vi "Tabelle zerlegen.vi"(11 "Tabelle":string[][](array[string])) -> (0 "Text":string[](array[string]), 1 "abschaltend":bool[](array[boolean]), 2 "quittieren?":bool[](array[boolean]), 3 "Ansprechverzögerung":dbl[](array[numeric]), 5 "max Nummer":i32)   [LabVIEW 2020, in "Stoerungen.lvlib"]
uses:
  Stoerungen.lvlib
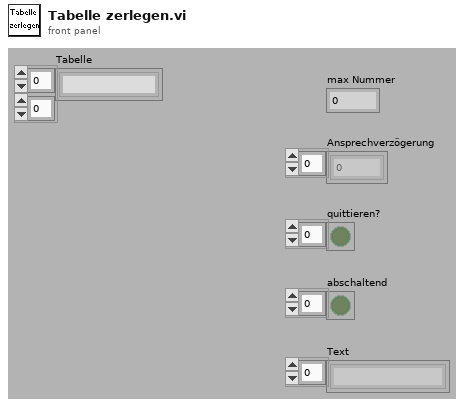
[diagram p1: front panel]
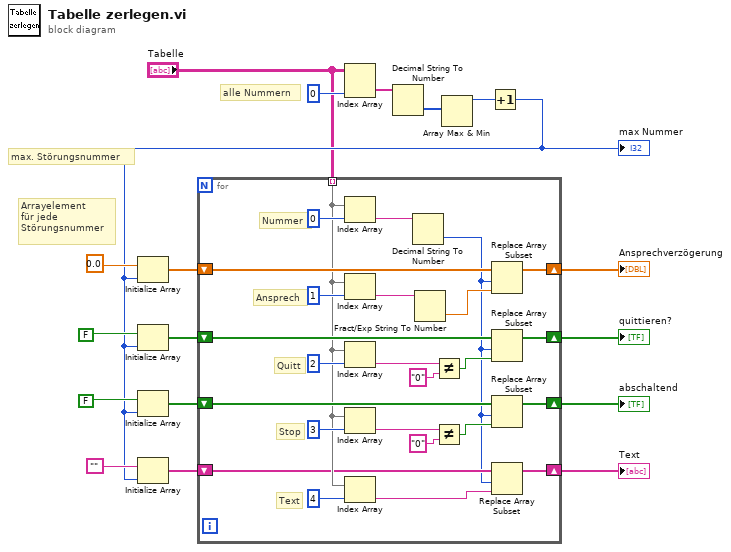
[diagram p0: block diagram]
diagram:
  # "Arrayelement\nfür jede\nStörungsnummer"
  # "max. Störungsnummer"
  # "alle Nummern"
  n1 = Index Array(array="Tabelle", index (col)=0 ("Index")) -> (element=w13:string[])  [unwired: 1 in]
  n2 = Decimal String To Number(string=w13) -> (number=w12:i32[])  [unwired: 3 out]
  n3 = Array Max & Min(array=w12) -> (max value=w11:i32)  [unwired: 3 out]
  n4 = Increment(x=w11) -> (x+1=w6:i32)
  "max Nummer" <- w6
  n5 = Initialize Array(0.0, w6) -> (w15:dbl[])
  n6 = Initialize Array(FALSE, w6) -> (w16:bool[])
  n7 = Initialize Array(FALSE, w6) -> (w10:bool[])
  n8 = Initialize Array("", w6) -> (w8:string[])
  n9 = for {
    shift-right: [w43] -> w4
    shift-left: w16 -> [w42]
    shift-right: [w40] -> w5
    shift-left: w15 -> [w41]
    tunnel: "Tabelle" -> [w23] mode=indexing
    shift-right: [w26] -> w3
    shift-left: w10 -> [w27]
    shift-right: [w22] -> w2
    shift-left: w8 -> [w21]
    # "Text"
    # "Stop"
    # "Quitt"
    # "Ansprech"
    # "Nummer"
    n10 = Index Array(array=w23, index=0 ("Index")) -> (element=w34:string)
    n11 = Index Array(array=w23, index=1 ("Index")) -> (element=w32:string)
    n12 = Index Array(array=w23, index=2 ("Index")) -> (element=w36:string)
    n13 = Index Array(array=w23, index=3 ("Index")) -> (element=w30:string)
    n14 = Index Array(array=w23, index=4 ("Index")) -> (element=w20:string)
    n15 = Decimal String To Number(string=w34) -> (number=w19:i32)  [unwired: 3 out]
    n16 = Fract/Exp String To Number(string=w32) -> (number=w31:dbl)  [unwired: 4 out]
    n17 = Not Equal?(x=w36, y="0") -> (x != y?=w39:bool)
    n18 = Not Equal?(x=w30, y="0") -> (x != y?=w28:bool)
    n19 = Replace Array Subset(array=w41, new element=w31, index=w19) -> (w40:dbl[])
    n20 = Replace Array Subset(array=w42, new element=w39, index=w19) -> (w43:bool[])
    n21 = Replace Array Subset(array=w27, new element=w28, index=w19) -> (w26:bool[])
    n22 = Replace Array Subset(array=w21, new element=w20, index=w19) -> (w22:string[])
  }
  "Ansprechverzögerung" <- w5
  "quittieren?" <- w4
  "abschaltend" <- w3
  "Text" <- w2
